vi "FindIntersectionOfRectangles2.vi"(10 "Wire":T1, 11 "Node":T1) -> (3 "Intersect?":bool)   [LabVIEW 2014]
uses:
  <vilib>/Utility/miscctls.llb/LVRectTypeDef.ctl
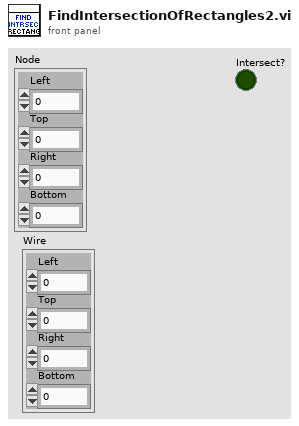
[diagram p1: front panel]
types:
  T1 = typedef "LVRectTypeDef.ctl" = cluster{"Left":i16, "Top":i16, "Right":i16, "Bottom":i16}
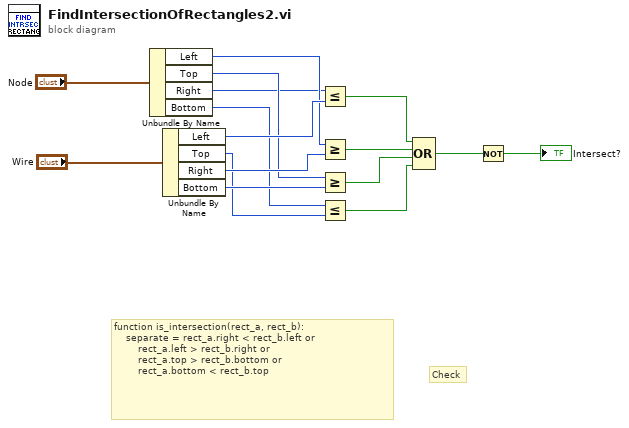
[diagram p0: block diagram]
diagram:
  # "Check"
  # "function is_intersection(rect_a, rect_b):\n    separate = rect_a.right < rect_b.left or\n        rect_a.left > rect_b.right or\n        rect_a.top > rect_b.bottom or\n        rect_a.bottom < rect_b.top"
  n1 = Unbundle By Name("Node") -> ("Left"=w4:i16, "Top"=w3:i16, "Right"=w2:i16, "Bottom"=w1:i16)
  n2 = Unbundle By Name("Wire") -> ("Left"=w13:i16, "Top"=w14:i16, "Right"=w16:i16, "Bottom"=w15:i16)
  n3 = Less Or Equal?(x=w2, y=w13) -> (x <= y?=w11:bool)
  n4 = Greater Or Equal?(x=w4, y=w16) -> (x >= y?=w7:bool)
  n5 = Greater Or Equal?(x=w3, y=w15) -> (x >= y?=w10:bool)
  n6 = Less Or Equal?(x=w1, y=w14) -> (x <= y?=w9:bool)
  n7 = Compound Arithmetic op=OR(w11, w7, w10, w9) -> (w12:bool)
  n8 = Not(x=w12) -> (.not. x?=→"Intersect?":bool)
